vi "ttm_variableCalculator_poller.vi"() -> ()   [LabVIEW 2010]
panel:
  out "rawTimeAfterRamp 2":dbl
  out "cycleamount":dbl
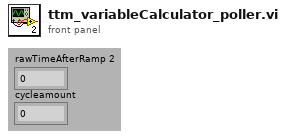
[diagram p1: front panel]
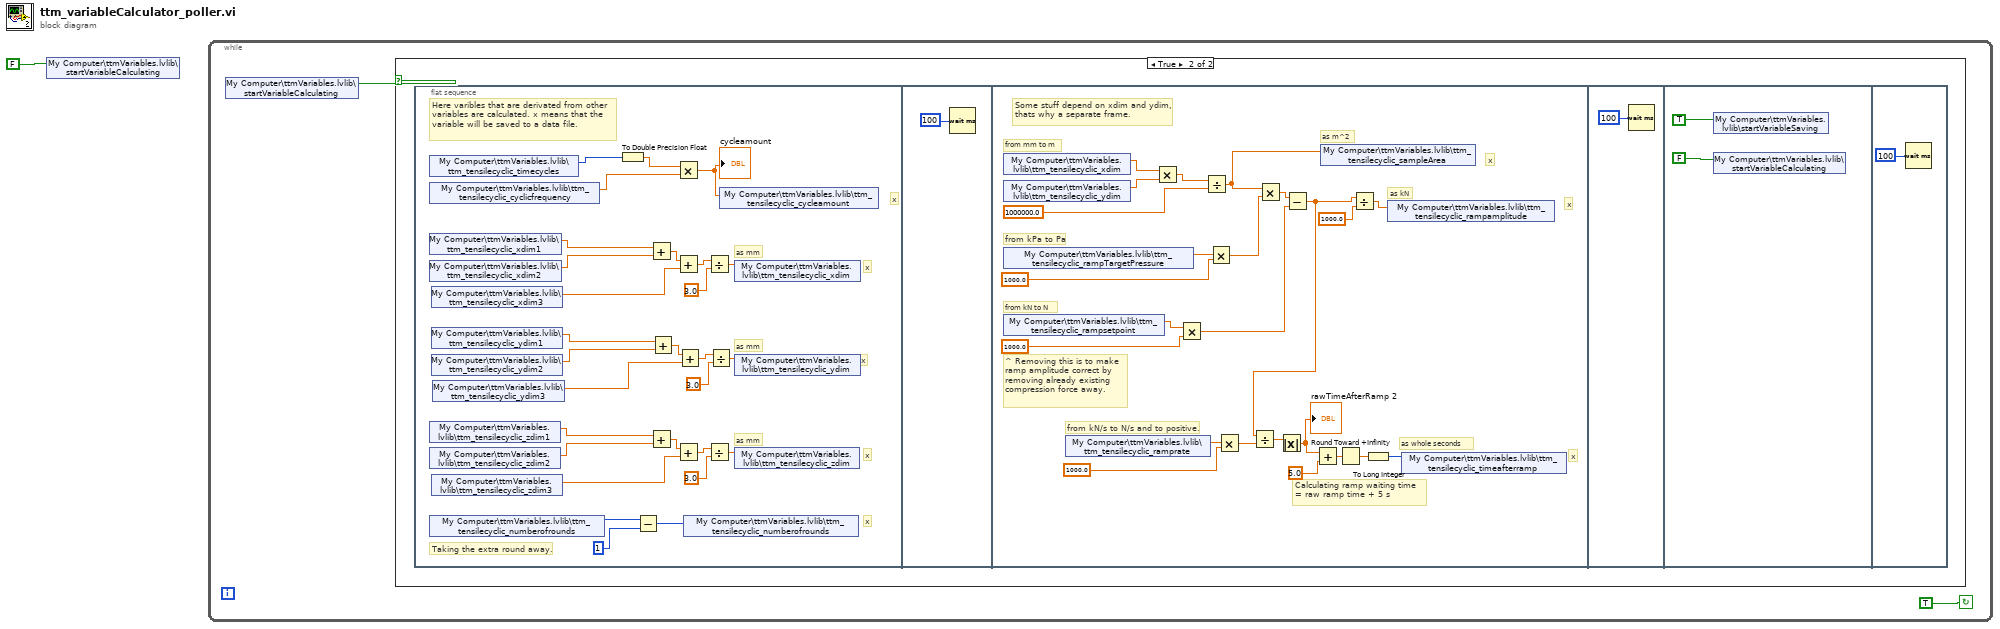
[diagram p0: block diagram]
diagram:
  n1 = shared-variable "My Computer\\ttmVariables.lvlib\\startVariableCalculating"(FALSE ("startLogging")) -> ()  [unwired: 1 in, 1 out]
  n2 = while {
    stop <- TRUE continue-if-true
    n3 = shared-variable "My Computer\\ttmVariables.lvlib\\startVariableCalculating"() -> (w3:bool)  [unwired: 1 in, 1 out]
    n4 = case shown="True" w3 {
      frame False {
      }
      frame True {
        n5 = flat-sequence {
          frame #0 {
            # "Taking the extra round away."
            # "x"
            # "as mm"
            # "as mm"
            # "as mm"
            # "x"
            # "x"
            # "x"
            # "x"
            # "Here varibles that are derivated from other variables are calculated. x means that the variable will be saved to a data file."
            n6 = shared-variable "My Computer\\ttmVariables.lvlib\\ttm_tensilecyclic_timecycles"() -> (w29:i32)  [unwired: 1 in, 1 out]
            n7 = shared-variable "My Computer\\ttmVariables.lvlib\\ttm_tensilecyclic_cyclicfrequency"() -> (w31:dbl)  [unwired: 1 in, 1 out]
            n8 = shared-variable "My Computer\\ttmVariables.lvlib\\ttm_tensilecyclic_xdim1"() -> (w27:dbl)  [unwired: 1 in, 1 out]
            n9 = shared-variable "My Computer\\ttmVariables.lvlib\\ttm_tensilecyclic_xdim2"() -> (w25:dbl)  [unwired: 1 in, 1 out]
            n10 = shared-variable "My Computer\\ttmVariables.lvlib\\ttm_tensilecyclic_zdim1"() -> (w13:dbl)  [unwired: 1 in, 1 out]
            n11 = shared-variable "My Computer\\ttmVariables.lvlib\\ttm_tensilecyclic_zdim2"() -> (w11:dbl)  [unwired: 1 in, 1 out]
            n12 = shared-variable "My Computer\\ttmVariables.lvlib\\ttm_tensilecyclic_numberofrounds"() -> (w5:i32)  [unwired: 1 in, 1 out]
            n13 = shared-variable "My Computer\\ttmVariables.lvlib\\ttm_tensilecyclic_xdim3"() -> (w24:dbl)  [unwired: 1 in, 1 out]
            n14 = shared-variable "My Computer\\ttmVariables.lvlib\\ttm_tensilecyclic_ydim1"() -> (w20:dbl)  [unwired: 1 in, 1 out]
            n15 = shared-variable "My Computer\\ttmVariables.lvlib\\ttm_tensilecyclic_ydim2"() -> (w18:dbl)  [unwired: 1 in, 1 out]
            n16 = shared-variable "My Computer\\ttmVariables.lvlib\\ttm_tensilecyclic_zdim3"() -> (w10:dbl)  [unwired: 1 in, 1 out]
            n17 = shared-variable "My Computer\\ttmVariables.lvlib\\ttm_tensilecyclic_ydim3"() -> (w17:dbl)  [unwired: 1 in, 1 out]
            n18 = To Double Precision Float(number=w29) -> (double precision float=w30:dbl)
            n19 = Subtract(x=w5, y=1) -> (x-y=w6:i32)
            n20 = Add(x=w27, y=w25) -> (x+y=w26:dbl)
            n21 = Add(x=w13, y=w11) -> (x+y=w12:dbl)
            n22 = Add(x=w20, y=w18) -> (x+y=w19:dbl)
            n23 = Multiply(x=w30, y=w31) -> (x*y=w28:dbl)
            "cycleamount" <- w28
            n24 = Add(x=w26, y=w24) -> (x+y=w23:dbl)
            n25 = Add(x=w12, y=w10) -> (x+y=w9:dbl)
            n26 = Add(x=w19, y=w17) -> (x+y=w16:dbl)
            n27 = shared-variable "My Computer\\ttmVariables.lvlib\\ttm_tensilecyclic_numberofrounds"(w6) -> ()  [unwired: 1 in, 1 out]
            n28 = Divide(x=w23, y=3.0) -> (x/y=w21:dbl)
            n29 = Divide(x=w9, y=3.0) -> (x/y=w7:dbl)
            n30 = Divide(x=w16, y=3.0) -> (x/y=w14:dbl)
            n31 = shared-variable "My Computer\\ttmVariables.lvlib\\ttm_tensilecyclic_cycleamount"(w28) -> ()  [unwired: 1 in, 1 out]
            n32 = shared-variable "My Computer\\ttmVariables.lvlib\\ttm_tensilecyclic_xdim"(w21) -> ()  [unwired: 1 in, 1 out]
            n33 = shared-variable "My Computer\\ttmVariables.lvlib\\ttm_tensilecyclic_ydim"(w14) -> ()  [unwired: 1 in, 1 out]
            n34 = shared-variable "My Computer\\ttmVariables.lvlib\\ttm_tensilecyclic_zdim"(w7) -> ()  [unwired: 1 in, 1 out]
          }
          frame #1 {
            n35 = Wait (ms)(milliseconds to wait=u32 100) -> ()  [unwired: 1 out]
          }
          frame #2 {
            # "Some stuff depend on xdim and ydim, thats why a separate frame."
            # "from kN/s to N/s and to positive."
            # "from kN to N"
            # "from mm to m"
            # "from kPa to Pa"
            # "as whole seconds"
            # "^ Removing this is to make ramp amplitude correct by removing already existing compression force away."
            # "x"
            # "Calculating ramp waiting time = raw ramp time + 5 s"
            # "x"
            # "x"
            # "as kN"
            # "as m^2"
            n36 = shared-variable "My Computer\\ttmVariables.lvlib\\ttm_tensilecyclic_xdim"() -> (w50:dbl)  [unwired: 1 in, 1 out]
            n37 = shared-variable "My Computer\\ttmVariables.lvlib\\ttm_tensilecyclic_ydim"() -> (w51:dbl)  [unwired: 1 in, 1 out]
            n38 = shared-variable "My Computer\\ttmVariables.lvlib\\ttm_tensilecyclic_rampTargetPressure"() -> (w40:dbl)  [unwired: 1 in, 1 out]
            n39 = shared-variable "My Computer\\ttmVariables.lvlib\\ttm_tensilecyclic_rampsetpoint"() -> (w54:dbl)  [unwired: 1 in, 1 out]
            n40 = shared-variable "My Computer\\ttmVariables.lvlib\\ttm_tensilecyclic_ramprate"() -> (w38:dbl)  [unwired: 1 in, 1 out]
            n41 = Multiply(x=w50, y=w51) -> (x*y=w43:dbl)
            n42 = Multiply(x=w54, y=1000.0) -> (x*y=w53:dbl)
            n43 = Divide(x=w43, y=1000000.0) -> (x/y=w52:dbl)
            n44 = Multiply(x=w40, y=1000.0) -> (x*y=w41:dbl)
            n45 = Multiply(x=w38, y=1000.0) -> (x*y=w36:dbl)
            n46 = Multiply(x=w52, y=w41) -> (x*y=w49:dbl)
            n47 = Subtract(x=w49, y=w53) -> (x-y=w33:dbl)
            n48 = Divide(x=w33, y=w36) -> (x/y=w34:dbl)
            n49 = Absolute Value(x=w34) -> (abs(x)=w35:dbl)
            "rawTimeAfterRamp 2" <- w35
            n50 = Add(x=w35, y=5.0) -> (x+y=w46:dbl)
            n51 = shared-variable "My Computer\\ttmVariables.lvlib\\ttm_tensilecyclic_sampleArea"(w52) -> ()  [unwired: 1 in, 1 out]
            n52 = Round Toward +Infinity(x=w46) -> (ceil(x): smallest int >= x=w47:dbl)
            n53 = Divide(x=w33, y=1000.0) -> (x/y=w55:dbl)
            n54 = To Long Integer(number=w47) -> (32bit integer=w48:i32)
            n55 = shared-variable "My Computer\\ttmVariables.lvlib\\ttm_tensilecyclic_rampamplitude"(w55) -> ()  [unwired: 1 in, 1 out]
            n56 = shared-variable "My Computer\\ttmVariables.lvlib\\ttm_tensilecyclic_timeafterramp"(w48) -> ()  [unwired: 1 in, 1 out]
          }
          frame #3 {
            n57 = Wait (ms)(milliseconds to wait=u32 100) -> ()  [unwired: 1 out]
          }
          frame #4 {
            n58 = shared-variable "My Computer\\ttmVariables.lvlib\\startVariableSaving"(TRUE ("startLogging")) -> ()  [unwired: 1 in, 1 out]
            n59 = shared-variable "My Computer\\ttmVariables.lvlib\\startVariableCalculating"(FALSE ("startLogging")) -> ()  [unwired: 1 in, 1 out]
          }
          frame #5 {
            n60 = Wait (ms)(milliseconds to wait=u32 100) -> ()  [unwired: 1 out]
          }
        }
      }
    }
  }
